vi "test_FrameEditor.vi"() -> ()   [LabVIEW 2020]
uses:
  Frame Configuration/FrameEditor.lvlib
panel:
  in  "Input File":path
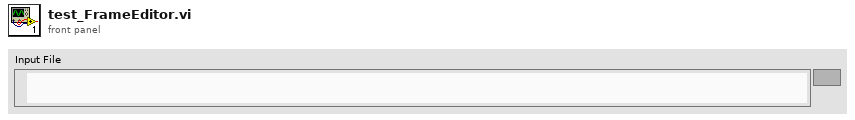
[diagram p1: front panel]
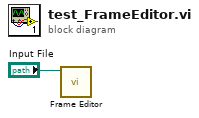
[diagram p0: block diagram]
diagram:
  n1 = call "Frame Editor.vi"("Input File"="Input File") -> ()  [unwired: 7 in, 4 out]
